vi "动态调用与子面板.vi"() -> ()   [LabVIEW 2013]
panel:
  in  "选择噪声":enum16{"高斯噪声", "均匀白噪声"}(ring)
  in  "停止":bool
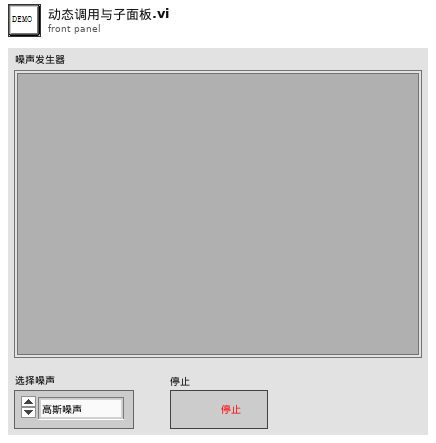
[diagram p1: front panel]
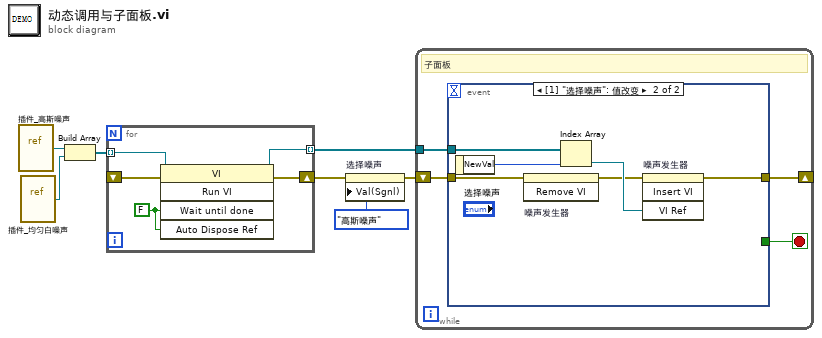
[diagram p0: block diagram]
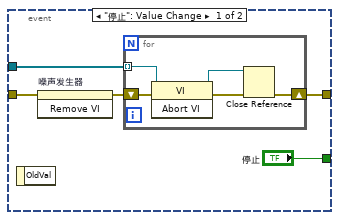
[diagram p2: hidden frame]
diagram:
  n1 = vi-ref "插件_高斯噪声.vi"() -> (w7:refnum<vi>)
  n2 = vi-ref "插件_均匀白噪声.vi"() -> (w6:refnum<vi>)
  n3 = Build Array(w7, w6) -> (w3:refnum<vi>[])
  n4 = for {
    tunnel: w3 -> [w11] mode=indexing
    shift-right: [w10] -> w2
    shift-left: _ -> [w8]
    tunnel: [w9] -> w1 mode=indexing
    w12 = FALSE ("结束前等待")
    n5 = invoke class="VI" method="Run VI"(reference=w11, error in=w8, "Wait until done"=w12, "Auto Dispose Ref"=w12) -> (reference out=w9:refnum<vi>, error out=w10:errorcluster)  [unwired: 1 in, 3 out]
  }
  n6 = property on="选择噪声" class="Enum (严格)"(error in=w2, "Val(Sgnl)"=enum16{"高斯噪声", "均匀白噪声"}."高斯噪声" ("值(信号)")) -> (error out=w4:errorcluster)  [unwired: 1 in, 1 out]
  n7 = while {
    tunnel: w1 -> [w15]
    shift-right: [w13] -> _
    shift-left: w4 -> [w14]
    stop <- w16 stop-if-true
    # "子面板"
    n8 = event shown="[1] \"选择噪声\": 值改变" {
      selector: _ -> [_ _]
      dyn-events: _ -> [_ _]
      timeout: _ -> [_ _]
      tunnel: ["停止" _] -> w16
      tunnel: w15 -> [w19 w32]
      tunnel: w14 -> [w20 w31]
      tunnel: [w18 w30] -> w13
      event "停止": Value Change {
        n9 = event-data() -> ()  [unwired: 1 in, 1 out]
        n10 = invoke on="噪声发生器" class="子面板" method="Remove VI"(error in=w20) -> (error out=w17:errorcluster)  [unwired: 2 in, 2 out]
        n11 = for {
          tunnel: w19 -> [w26] mode=indexing
          shift-right: [w22] -> w18
          shift-left: w17 -> [w23]
          n12 = invoke class="VI" method="Abort VI"(reference=w26, error in=w23) -> (reference out=w25:refnum<vi>, error out=w24:errorcluster)  [unwired: 1 in, 1 out]
          n13 = Close Reference(reference=w25, error in (no error)=w24) -> (error out=w22:errorcluster)
        }
      }
      event "选择噪声": Value Change {
        n14 = event-data() -> ("NewVal"=w27:enum16{"高斯噪声", "均匀白噪声"})  [unwired: 1 in]
        n15 = invoke on="噪声发生器" class="子面板" method="Remove VI"(error in=w31) -> (error out=w28:errorcluster)  [unwired: 2 in, 2 out]
        n16 = Index Array(array=w32, index=w27) -> (element=w29:refnum<vi>)
        n17 = invoke on="噪声发生器" class="子面板" method="Insert VI"(error in=w28, "VI Ref"=w29) -> (error out=w30:errorcluster)  [unwired: 2 in, 3 out]
      }
    }
  }
